vi "QSM Q holder.vi"(11 "error in (no error)":errorcluster) -> (4 "Q":refnum<queue>, 15 "error out":errorcluster)   [LabVIEW 2011]
uses:
  QSM Main Data.ctl
  QSM State List.ctl
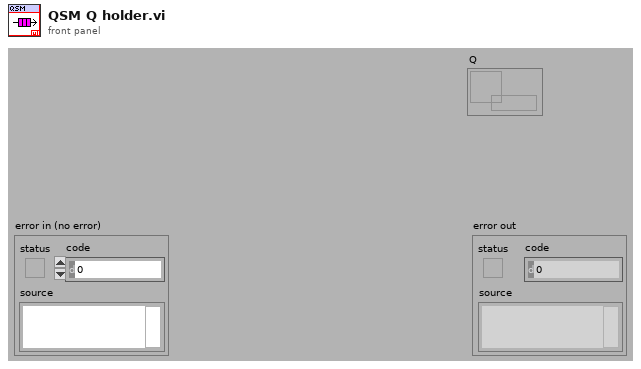
[diagram p1: front panel]
types:
  T1 = typedef "QSM Main Data.ctl" = cluster{"State":T2, "Var":variant}
  T2 = typedef "QSM State List.ctl" = enum16{"Idle", "Init <<<Start>>>", "Init Reg Controlers", "Init Stroker Ref FGV", "Init Driller Ref FGV", "Init Tractor Ref FGV", "Init All loops", "Init Mem Ctls", "Init GUI", "Init<<<End>>>", "Show options", "Options updated", "Show User Dialog", "User Updated", "Show About", "Show Help", "Debug Visibility", "End Application", "Mem Ctls", "Mem Graphs", "Post", "-------------", "Dialog Common Analog", "Chart Init", "Chart Var Selector Rings init", "Chart Read Settings from INI", "Chart Clear", "Chart Selection Changed", "Chart Time Changed", "Graph Dialog Show", "Annotation, New", "Annotation Created", "PCP CMD", "Show Welcome screen", "Dialog Tool analog", "Update PCP resistance", "Tool CMD", "Chart single autoscale", "Tool connenction state", "Show detailed view", "Sequences updated", "Show stroker wizard", "Change tool", "Reset Telemetry", "Update control units", "Stop Logging", "Start New Loggfile", "Log Init", "Copy INI files"}
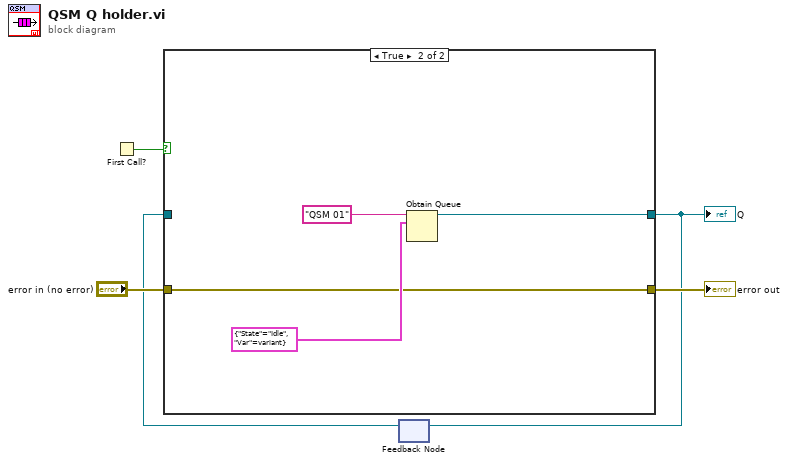
[diagram p0: block diagram]
diagram:
  n1 = First Call?() -> (First Call?: T/F=w3:bool)
  n2 = feedback #1() -> (w2:refnum<queue>)  [unwired: 1 in]
  n3 = case shown="True" w3 {
    tunnel: [w7 w8] -> w5
    tunnel: "error in (no error)" -> [w7 w8]
    tunnel: [w6 w11] -> w1
    tunnel: w2 -> [w6 _]
    frame False {
    }
    frame True {
      n4 = Obtain Queue(name (unnamed)="QSM 01", element data type=T1 {"State"=enum."Idle", "Var"=variant} ("Data")) -> (queue out=w11:refnum<queue>)  [unwired: 3 in, 2 out]
    }
  }
  "error out" <- w5
  "Q" <- w1
  n5 = feedback-in #1(w1) -> ()
